vi "SWT_CarT_0722.vi"() -> ()   [LabVIEW 2013]
uses:
  <vilib>/Utility/error.llb/DialogType.ctl
  <vilib>/DAQmx/write.llb/DAQmx Write (Analog DBL 1Chan 1Samp).vi
  <vilib>/DAQmx/create/channels.llb/DAQmx Create Channel (AO-Voltage-Basic).vi
  <vilib>/DAQmx/miscellaneous.llb/DAQmx Fill In Error Info.vi
panel:
  in  "RFP exp":dbl=1.35
  in  "GFP exp":dbl=1.35
  in  "BF exp":dbl=1.35
  in  "WF aquare":bool
  out "in TBD":bool
  in  "TBD":bool
  in  "Next":bool=TRUE
  in  "Delete":bool
  in  "index(1~n)":i32=17 min=-1 max=43 step=1
  out "yn":i32=32
  out "y pose":dbl=-0.987708848659002 format="%.4g"
  out "xn":i32=44
  out "x pose":dbl=1.0289425462047794 format="%.4g"
  out "TBD num":dbl=12.0
  out "Cell num":i32=60
  out "Total num":i32=2025
  in  "Coordinate Path":path=path "D:/20230823/WF/result.xlsx"
  in  "d WF":dbl=1.35
  in  "y WF":dbl=-1.3212
  in  "x WF":dbl=-2.141
  in  "Init":bool=TRUE
  in  "scan test":bool
  in  "Reset":bool
  out "备份细胞坐标数组(X,Y)":i32[][](array[numeric])=[[11, 43, 478, 478, 1], [4, 41, 428, 428, 1], [24, 45, 343, 343, 1], [27, 38, 342, 342, 1], [27, 19, 311, 311, 1], [36, 19, 306, 306, 1], [10, 42, 296, 329, 1], [23, 28, 291, 291, 1], [15, 22, 283, 283, 1], [9, 32, 261, 261, 1], [24, 23, 252, 280, 1], [37, 36, 251, 251, 1], [11, 38, 246, 246, 1], [27, 6, 245, 245, 1], [28, 42, 240, 240, 1], [40, 39, 240, 267, 1], [16, 23, 230, 230, 1], [15, 40, 228, 228, 1], [27, 34, 227, 227, 1], [27, 13, 225, 225, 1], [10, 32, 222, 222, 1], [11, 20, 208, 231, 1], [23, 19, 208, 208, 1], [21, 13, 204, 226, 1], [25, 21, 199, 199, 1], [21, 1, 199, 199, 1], [29, 2, 197, 197, 1], [23, 35, 193, 215, 1], [23, 43, 189, 189, 1], [8, 13, 188, 188, 1], [30, 42, 188, 188, 1], [16, 18, 183, 183, 1], [29, 22, 183, 183, 1], [14, 41, 181, 181, 1], [9, 19, 180, 180, 1], [37, 37, 179, 179, 1], [42, 13, 176, 176, 1], [16, 39, 171, 171, 1], [30, 12, 170, 189, 1], [17, 26, 168, 168, 1], [8, 28, 168, 187, 1], [40, 26, 167, 167, 1], [42, 29, 159, 159, 1], [15, 8, 159, 159, 1], [27, 28, 158, 176, 1], [17, 6, 154, 154, 1], [26, 26, 154, 154, 1], [18, 32, 150, 167, 1], [36, 33, 150, 150, 1], [9, 22, 147, 147, 1], [40, 36, 147, 147, 1], [35, 13, 146, 146, 1], [27, 11, 146, 146, 1], [24, 34, 145, 161, 1], [34, 26, 143, 159, 1], [28, 19, 143, 143, 1], [10, 16, 142, 142, 1], [24, 28, 139, 155, 1], [17, 23, 139, 154, 1], [19, 11, 136, 136, 1], [20, 23, 135, 135, 1], [44, 39, 133, 133, 1], [12, 16, 133, 148, 1], [38, 37, 133, 133, 1], [3, 26, 133, 133, 1], [32, 17, 133, 133, 1], [25, 20, 133, 133, 1], [24, 9, 131, 146, 1], [10, 22, 127, 127, 1], [43, 26, 127, 127, 1], [19, 36, 127, 127, 1], [14, 25, 125, 125, 1], [30, 34, 125, 139, 1], [10, 39, 124, 138, 1], [38, 36, 124, 124, 1], [5, 28, 123, 123, 1], [6, 32, 121, 121, 1], [28, 23, 120, 120, 1], [35, 26, 120, 120, 1], [28, 24, 119, 119, 1], [37, 35, 118, 118, 1], [11, 17, 117, 130, 1], [31, 21, 117, 117, 1], [29, 45, 117, 117, 1], [37, 29, 117, 117, 1], [41, 37, 116, 116, 1], [8, 26, 115, 128, 1], [15, 42, 115, 128, 1], [27, 27, 115, 115, 1], [14, 37, 115, 128, 1], [19, 10, 112, 112, 1], [35, 17, 110, 110, 1], [29, 38, 110, 110, 1], [37, 22, 110, 122, 1], [38, 7, 110, 110, 1], [28, 8, 109, 109, 1], [43, 25, 108, 108, 1], [26, 6, 107, 107, 1], [37, 15, 107, 107, 1], [10, 20, 106, 106, 1], [17, 44, 106, 106, 1], [44, 1, 106, 106, 1], [31, 41, 106, 106, 1], [20, 33, 106, 117, 1], [38, 20, 105, 105, 1], [40, 28, 105, 105, 1], [16, 34, 105, 105, 1], [33, 35, 105, 105, 1], [19, 26, 105, 105, 1], [11, 31, 105, 105, 1], [42, 19, 105, 105, 1], [24, 22, 105, 105, 1], [38, 28, 104, 104, 1], [42, 44, 104, 104, 1], [29, 19, 104, 104, 1], [30, 36, 104, 115, 1], [27, 12, 104, 104, 1], [27, 32, 103, 103, 1], [14, 34, 103, 103, 1], [27, 35, 102, 102, 1], [13, 20, 102, 113, 1], [39, 23, 101, 101, 1], [25, 26, 101, 101, 1], [19, 25, 101, 101, 1], [17, 31, 100, 100, 1], [24, 38, 100, 111, 1], [30, 23, 99, 110, 1], [11, 24, 99, 110, 1], [7, 39, 98, 109, 1], [10, 13, 98, 98, 1], [30, 26, 97, 97, 1], [32, 26, 97, 97, 1], [28, 21, 96, 107, 1], [40, 1, 96, 107, 1], [42, 25, 95, 95, 1], [4, 20, 95, 95, 1], [24, 27, 95, 95, 1], [43, 39, 94, 94, 1], [24, 40, 93, 104, 1], [6, 24, 92, 92, 1], [44, 35, 91, 101, 1], [4, 23, 91, 91, 1], [27, 18, 91, 101, 1], [26, 23, 91, 101, 1], [6, 26, 91, 91, 1], [27, 25, 90, 100, 1], [13, 31, 90, 90, 1], [1, 23, 90, 90, 1], [36, 9, 90, 90, 1], [15, 29, 89, 89, 1], [30, 31, 89, 89, 1], [25, 27, 89, 89, 1], [27, 31, 88, 88, 1], [15, 17, 88, 88, 1], [41, 10, 88, 88, 1], [11, 16, 87, 97, 1], [11, 40, 87, 87, 1], [43, 42, 87, 87, 1], [9, 34, 86, 86, 1], [35, 27, 86, 86, 1], [6, 34, 85, 85, 1], [24, 1, 84, 84, 1], [42, 36, 84, 84, 1], [23, 23, 84, 84, 1], [35, 22, 83, 83, 1], [30, 1, 83, 83, 1], [29, 4, 83, 83, 1], [3, 33, 83, 83, 1], [45, 6, 83, 83, 1], [20, 32, 82, 91, 1], [41, 17, 82, 91, 1], [39, 4, 82, 82, 1], [31, 36, 81, 81, 1], [45, 16, 81, 81, 1], [19, 17, 81, 89, 1], [24, 4, 80, 80, 1], [19, 33, 80, 80, 1], [21, 28, 80, 89, 1], [15, 9, 80, 80, 1], [4, 31, 80, 80, 1], [22, 7, 80, 80, 1], [41, 19, 79, 79, 1], [26, 24, 79, 79, 1], [18, 38, 79, 79, 1], [45, 11, 78, 78, 1], [19, 7, 78, 78, 1], [22, 16, 78, 78, 1], [31, 11, 78, 78, 1], [35, 10, 77, 77, 1], [28, 33, 77, 77, 1], [15, 35, 76, 85, 1], [28, 32, 76, 85, 1], [39, 26, 75, 75, 1], [26, 16, 75, 83, 1], [20, 1, 75, 83, 1], [6, 44, 75, 75, 1], [15, 21, 75, 75, 1], [28, 25, 75, 83, 1], [17, 5, 74, 74, 1], [41, 33, 74, 74, 1], [41, 21, 74, 74, 1], [25, 29, 74, 74, 1], [25, 2, 73, 73, 1], [6, 40, 73, 73, 1], [20, 26, 73, 81, 1], [45, 23, 73, 73, 1], [40, 37, 72, 80, 1], [30, 21, 72, 72, 1], [34, 34, 72, 80, 1], [9, 33, 72, 80, 1], [11, 4, 71, 71, 1], [16, 40, 71, 79, 1], [44, 32, 70, 70, 1], [20, 40, 70, 78, 1], [26, 20, 70, 78, 1], [41, 36, 70, 78, 1], [23, 12, 69, 69, 1], [22, 26, 69, 77, 1], [45, 21, 68, 68, 1], [25, 32, 68, 68, 1], [5, 29, 67, 67, 1], [23, 31, 67, 74, 1], [7, 41, 67, 74, 1], [27, 1, 67, 67, 1], [23, 32, 66, 74, 1], [35, 32, 66, 66, 1], [25, 16, 66, 73, 1], [18, 41, 66, 73, 1], [43, 5, 65, 65, 1], [14, 17, 65, 72, 1], [21, 43, 65, 65, 1], [28, 3, 65, 65, 1], [21, 7, 64, 64, 1], [14, 21, 63, 70, 1], [19, 23, 63, 70, 1], [24, 32, 62, 62, 1], [16, 20, 61, 61, 1], [5, 38, 60, 60, 1], [22, 32, 59, 66, 1], [15, 34, 59, 59, 1], [11, 32, 57, 63, 1], [8, 44, 56, 63, 1], [34, 21, 55, 61, 1], [29, 35, 52, 58, 1]]
  out "missing":i32[][](array[numeric])
  out "缺失坐标数":i32
  in  "Period 2/min":dbl
  in  "Repeat 2":dbl
  in  "Interval/ms":dbl=10.0
  in  "Offste/V":dbl=-1.0
  in  "Frame rate/Hz":dbl=50.0
  in  "Offset2/V":dbl=0.804
  in  "Volume num":dbl=360.0
  in  "slice par stack":dbl=120.0
  in  "step/um":dbl=0.6
  out "细胞坐标数组(X,Y)":i32[][](array[numeric])=[[27, 34, 227, 227, 1], [21, 13, 204, 226, 1], [29, 2, 197, 197, 1], [30, 42, 188, 188, 1], [9, 22, 147, 147, 1], [6, 32, 121, 121, 1], [28, 8, 109, 109, 1], [14, 34, 103, 103, 1], [27, 35, 102, 102, 1], [41, 19, 79, 79, 1], [39, 26, 75, 75, 1], [6, 44, 75, 75, 1], [41, 21, 74, 74, 1], [20, 26, 73, 81, 1], [34, 34, 72, 80, 1], [11, 4, 71, 71, 1], [44, 32, 70, 70, 1], [20, 40, 70, 78, 1], [26, 20, 70, 78, 1], [41, 36, 70, 78, 1], [23, 12, 69, 69, 1], [22, 26, 69, 77, 1], [45, 21, 68, 68, 1], [25, 32, 68, 68, 1], [5, 29, 67, 67, 1], [23, 31, 67, 74, 1], [7, 41, 67, 74, 1], [27, 1, 67, 67, 1], [23, 32, 66, 74, 1], [35, 32, 66, 66, 1], [25, 16, 66, 73, 1], [18, 41, 66, 73, 1], [43, 5, 65, 65, 1], [14, 17, 65, 72, 1], [21, 43, 65, 65, 1], [28, 3, 65, 65, 1], [21, 7, 64, 64, 1], [14, 21, 63, 70, 1], [19, 23, 63, 70, 1], [24, 32, 62, 62, 1], [16, 20, 61, 61, 1], [5, 38, 60, 60, 1], [22, 32, 59, 66, 1], [15, 34, 59, 59, 1], [11, 32, 57, 63, 1], [8, 44, 56, 63, 1], [34, 21, 55, 61, 1], [29, 35, 52, 58, 1], [15, 40, 228, 228, 1], [26, 26, 154, 154, 1], [20, 23, 135, 135, 1], [24, 38, 100, 111, 1], [4, 41, 428, 428, 1], [24, 45, 343, 343, 1], [23, 43, 189, 189, 1], [18, 32, 150, 167, 1], [29, 45, 117, 117, 1], [19, 26, 105, 105, 1], [30, 36, 104, 115, 1], [41, 17, 82, 91, 1]]
  in  "x2 index":i32=41 min=1 max=45 step=1
  in  "y2 index":i32=41 min=1 max=45 step=1
  in  "y1 index":i32=1 min=1 max=45 step=1
  in  "x1 index":i32=5 min=1 max=45 step=1
  in  "y2":dbl=-1.7723000000000002 format="%.4f"
  in  "x2":dbl=0.7769500000000003 format="%.4f"
  in  "y1":dbl=1.811900000000001 format="%.4f"
  in  "x1":dbl=-2.4755499999999997 format="%.4f"
  in  "y to end":bool=TRUE
  in  "y to start":bool
  in  "x to end":bool=TRUE
  in  "x step forward":bool
  in  "x to start":bool=TRUE
  in  "x step backward":bool
  in  "y step backward":bool=TRUE
  in  "y step forward":bool
  out "芯片角点坐标":T1={"x1"=-2.4755499999999997, "y1"=1.811900000000001, "x2"=0.7769500000000003, "y2"=-1.7723000000000002, "x1 index"=5, "y1 index"=1, "x2 index"=41, "y2 index"=41, array2025x7[14175 elements], "missing"=[]}
  out "模板孔坐标数组":dbl[][](array[numeric])
  in  "Scanner":dbl(slide)=45.99999999999999 min=-50.0 max=150.0 step=1.0 scale=0.0..100.0
  out "finish":bool
  out "running":bool
  in  "Chanber num":dbl=17.0
  out "photo number":dbl
  in  "Period/min":dbl
  in  "Repeat":dbl=1.0
  in  "finish":bool=TRUE
  # "HUST WZF\n2023.08.20"
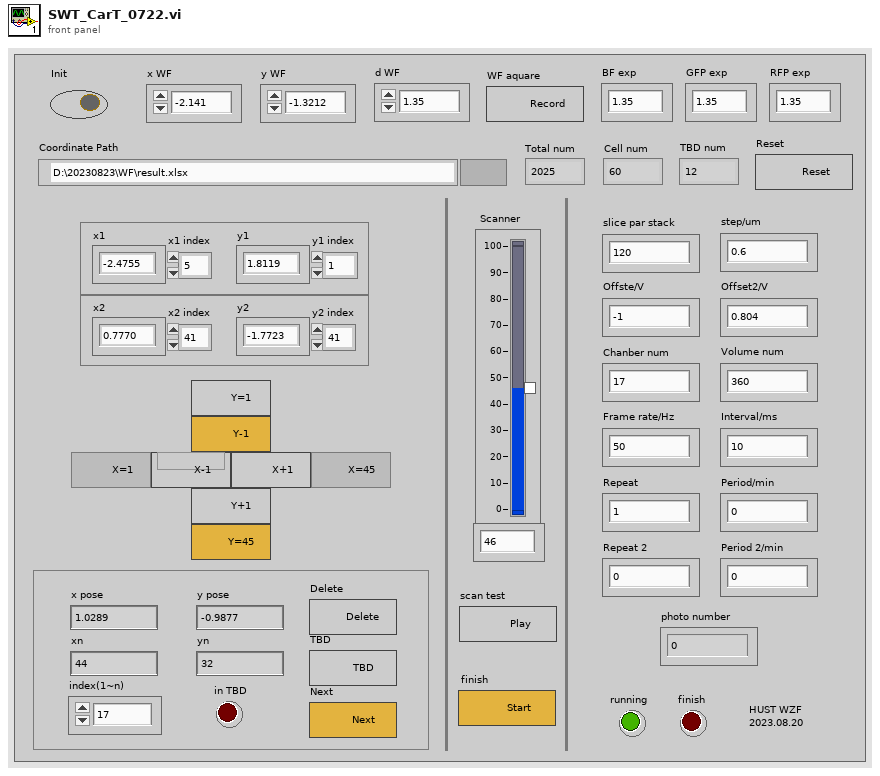
[diagram p1: front panel]
types:
  T1 = cluster{"x1":dbl, "y1":dbl, "x2":dbl, "y2":dbl, "x1 index":i32, "y1 index":i32, "x2 index":i32, "y2 index":i32, dbl[][], "missing":i32[][]}
  T2 = typedef "DialogType.ctl" = u16
  T3 = cluster{"x WF":dbl, "y WF":dbl, "d WF":dbl, "x1 index":i32, "y1 index":i32, "x2 index":i32, "y2 index":i32, dbl[][]}
  T4 = cluster{"y2":dbl, "y2":dbl, "y2":dbl, "y2":dbl, "x1 index":i32, "y1 index":i32, "x2 index":i32, "y2 index":i32, dbl[][], i32[][]}
  T5 = enum8{"Enabled", "Disabled", "Disabled and Grayed Out"}
  T6 = cluster{"x1":dbl, "y1":dbl, "x2":dbl, "y2":dbl, "x1 index":i32, "y1 index":i32, "x2 index":i32, "y2 index":i32, "模板孔坐标数组":dbl[][], "missing":i32[][]}
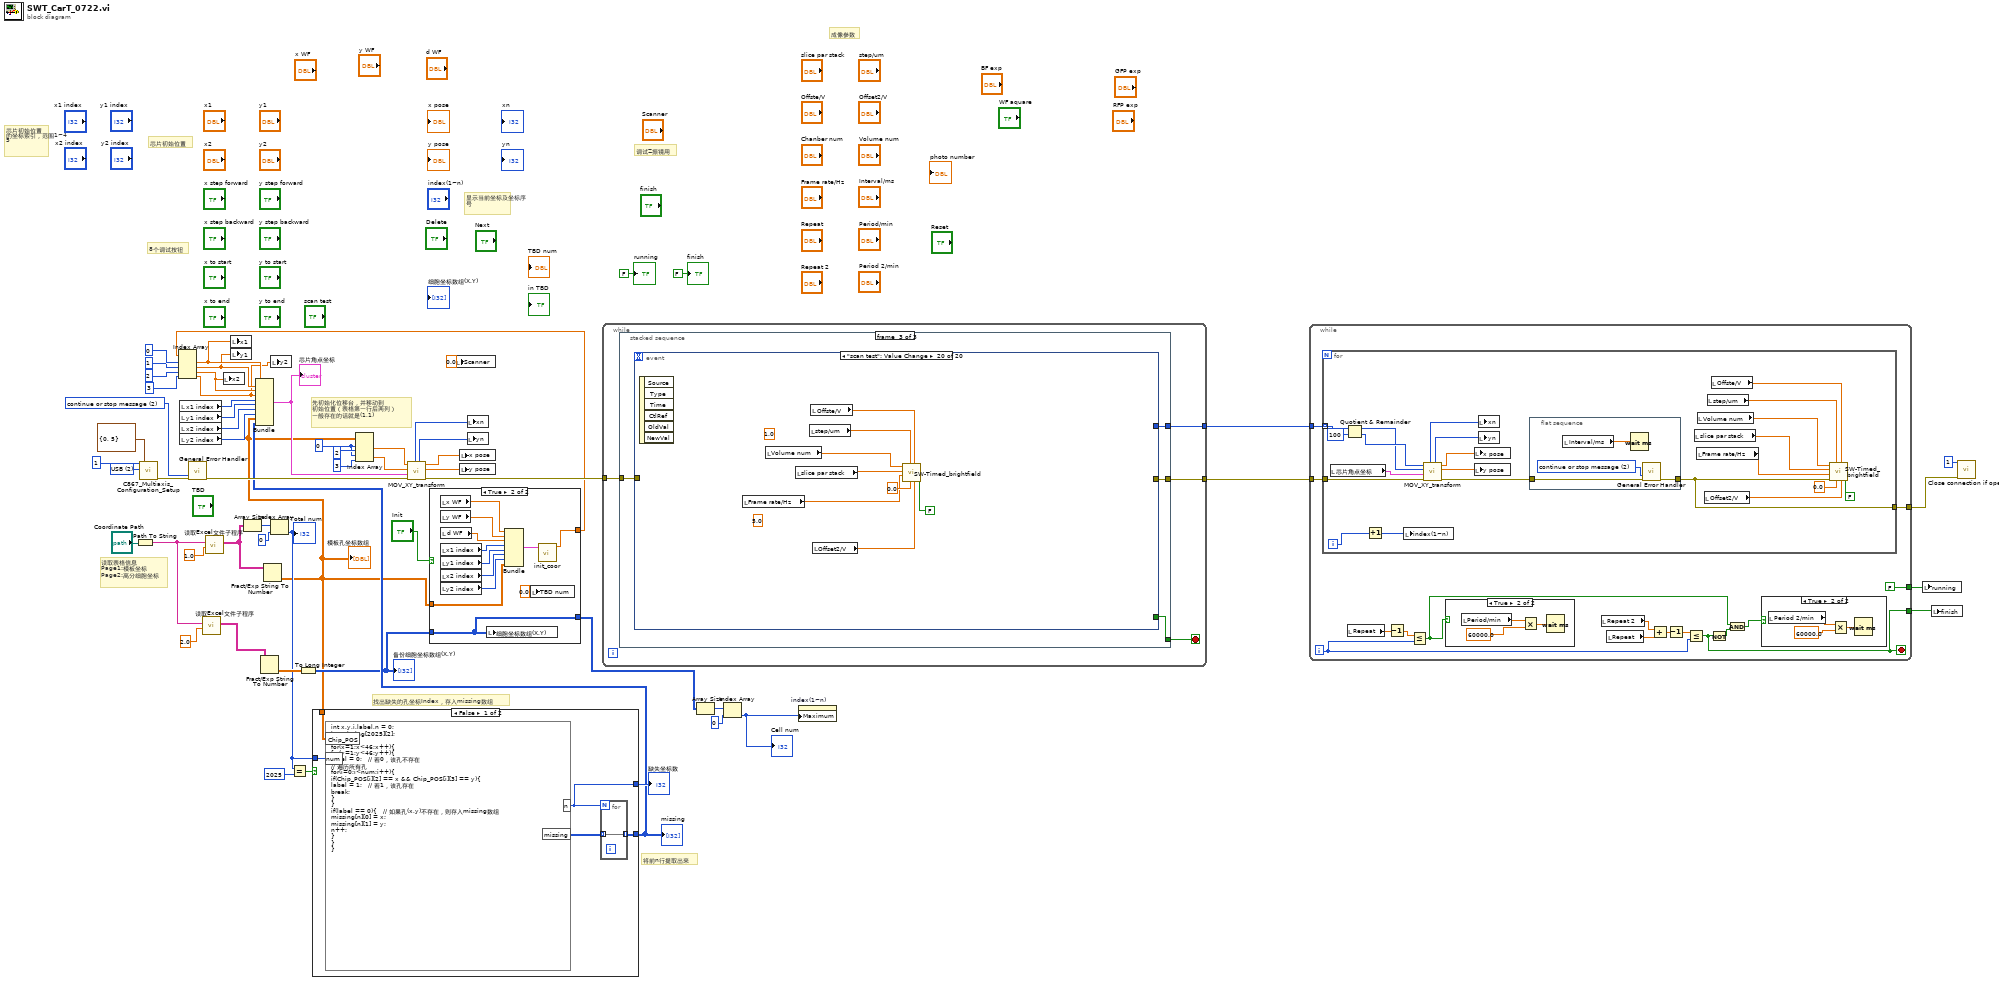
[diagram p0: block diagram]
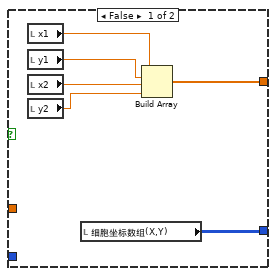
[diagram p2: hidden frame]
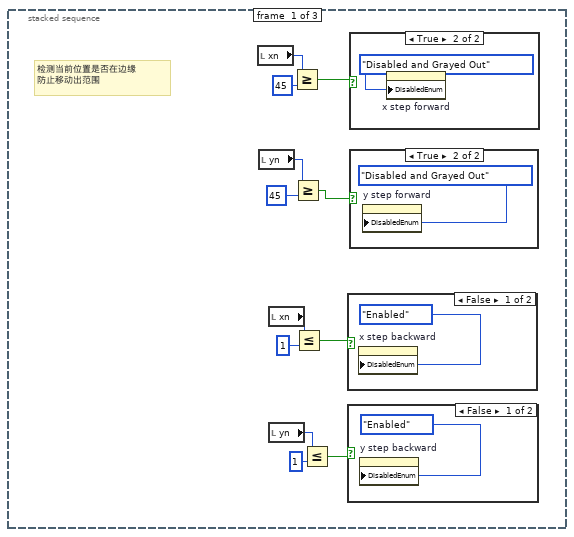
[diagram p5: hidden frame]
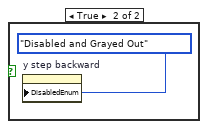
[diagram p6: hidden frame]
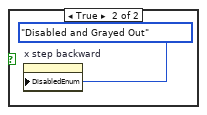
[diagram p7: hidden frame]
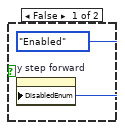
[diagram p8: hidden frame]
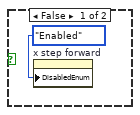
[diagram p9: hidden frame]
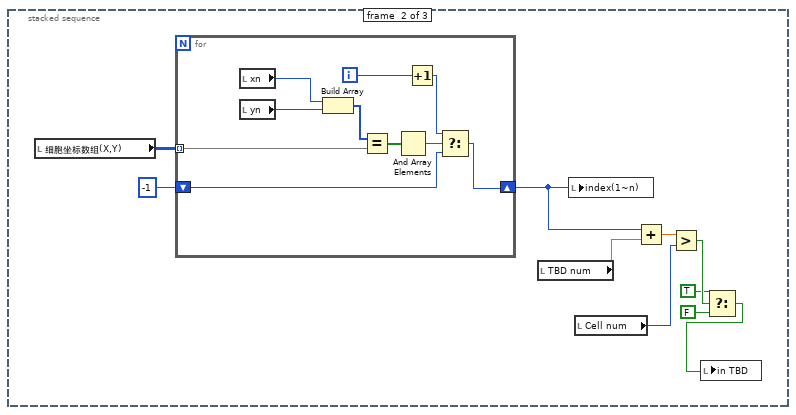
[diagram p10: hidden frame]
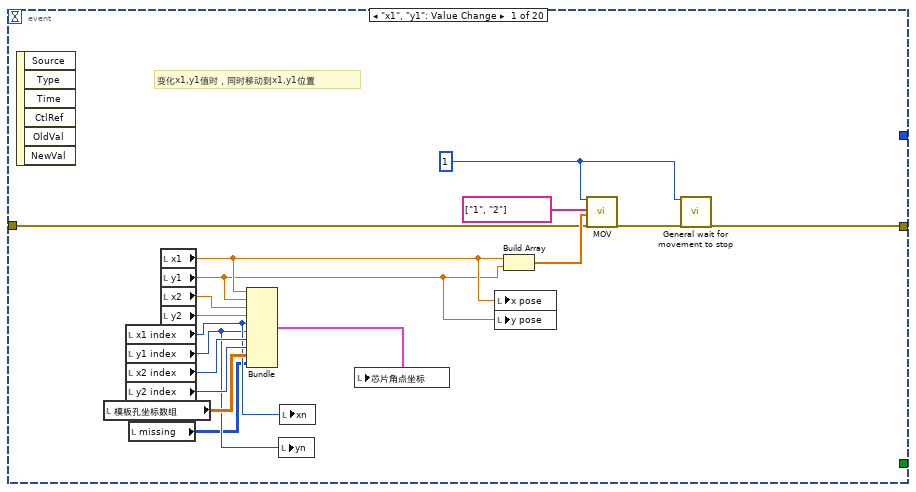
[diagram p11: hidden frame]
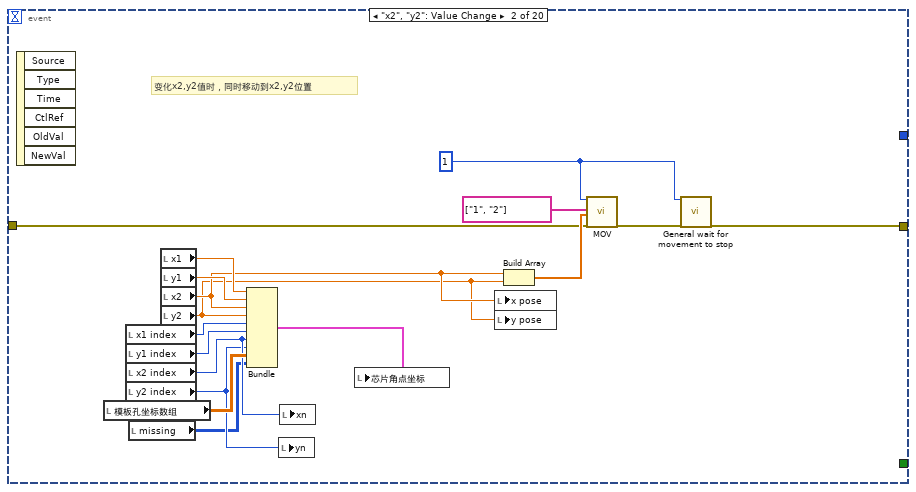
[diagram p12: hidden frame]
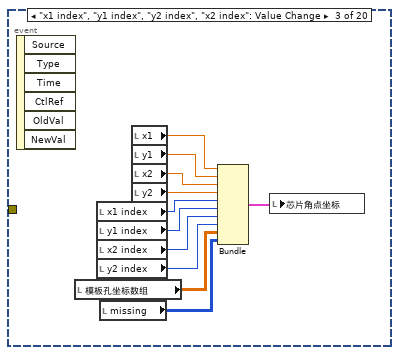
[diagram p13: hidden frame]
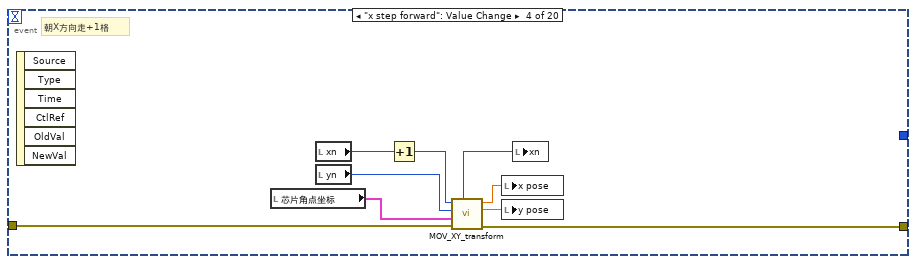
[diagram p14: hidden frame]
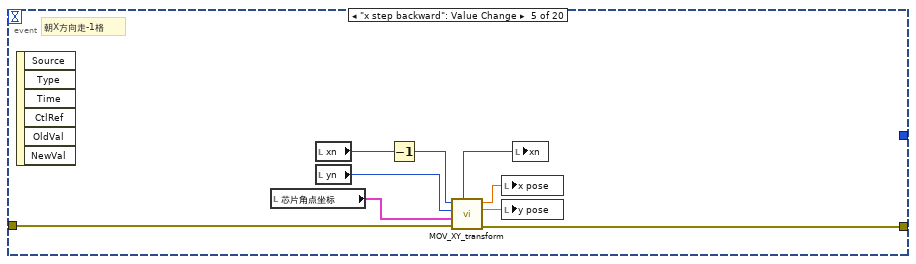
[diagram p15: hidden frame]
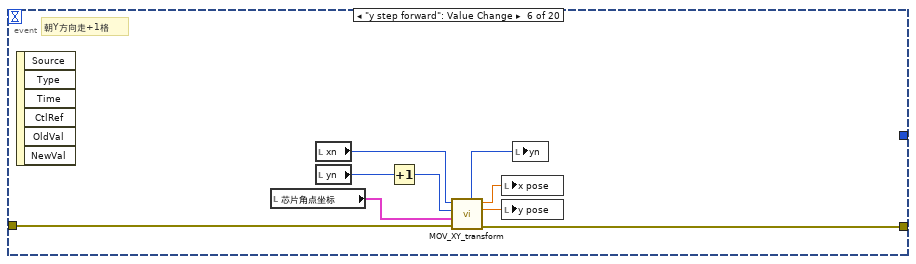
[diagram p16: hidden frame]
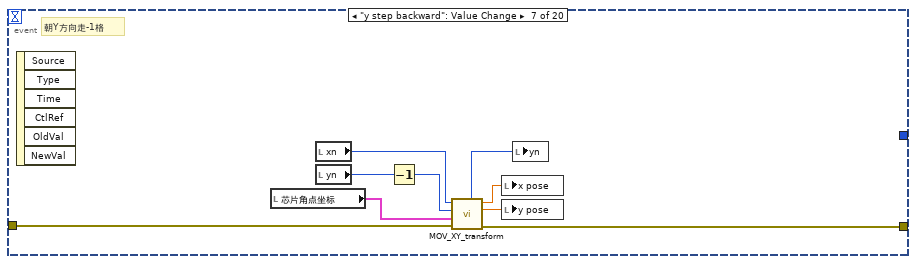
[diagram p17: hidden frame]
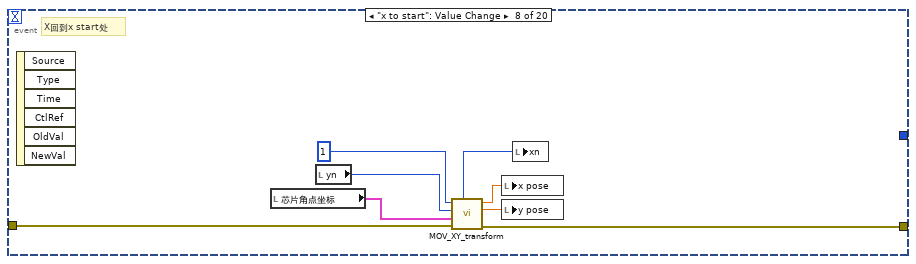
[diagram p18: hidden frame]
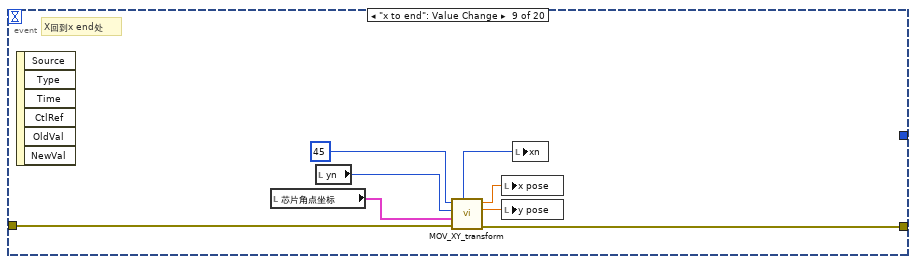
[diagram p19: hidden frame]
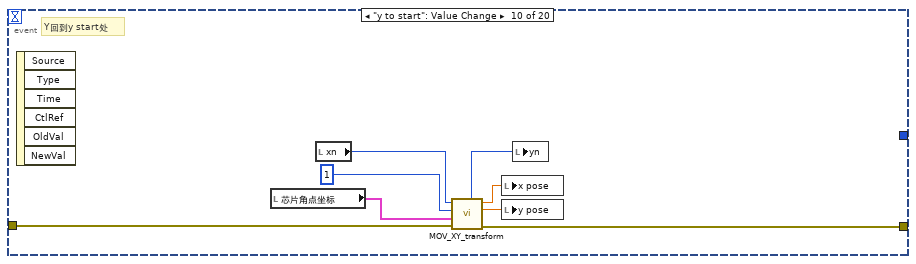
[diagram p20: hidden frame]
diagram:
  w18 = 0 ("索引 (行)")
  w53 = T2 2 items=["no dialog", "OK message", "continue or stop message", "OK message + warnings", "continue/stop + warnings"] ("type of dialog (OK msg:1)")
  w57 = u16 2 items=["RS232", "RS232 DaisyChain", "USB"] ("Interface")
  # "将前n行提取出来"
  # "找出缺失的孔坐标Index，存入missing数组"
  # "读取表格信息\nPage1:模板坐标\nPage2:高分细胞坐标"
  # "芯片初始位置\n的坐标索引，范围1~45"
  # "先初始化位移台，并移动到\n初始位置（表格第一行后两列）\n一般存在的话就是(1,1)"
  # "芯片初始位置"
  # "显示当前坐标及坐标序号"
  # "调试Z振镜用"
  # "8个调试按钮"
  # "成像参数"
  n1 = Path To String(path="Coordinate Path") -> (string=w39:string)
  n2 = call "C867_Multiaxis_Configuration_Setup.vi"("System no."=1, "Interface"=w57, "RS232 settings"=cluster{"Portnumber":i32, "Baudrate":u16} {"Portnumber"=0, "Baudrate"=5}) -> ("error out"=w54:errorcluster)  [unwired: 10 in, 6 out]
  n3 = local read "x1 index"() -> (w48:i32)
  n4 = local read "y1 index"() -> (w47:i32)
  n5 = local read "x2 index"() -> (w46:i32)
  n6 = local read "y2 index"() -> (w45:i32)
  n7 = call <vilib>:"General Error Handler.vi"("type of dialog (OK msg:1)"=w53, "error in (no error)"=w54) -> ("error out"=w52:errorcluster)  [unwired: 9 in, 4 out]
  n8 = call "读取Excel文件子程序.vi"("页"=2.0, "Filename"=w39) -> ("数据"=w42:string[][])  [unwired: 8 in, 1 out]
  n9 = call "读取Excel文件子程序.vi"("页"=1.0, "Filename"=w39) -> ("数据"=w43:string[][])  [unwired: 8 in, 1 out]
  n10 = Array Size(array=w43) -> (size(s)=w50:i32[])
  n11 = Fract/Exp String To Number(string=w42) -> (number=w37:dbl[][])  [unwired: 3 in, 1 out]
  n12 = Fract/Exp String To Number(string=w43) -> (number=w6:dbl[][])  [unwired: 3 in, 1 out]
  "模板孔坐标数组" <- w6
  n13 = Index Array(array=w50, index=0 ("索引")) -> (element=w34:i32)
  "Total num" <- w34
  n14 = Equal?(x=w34, y=2025) -> (x = y?=w36:bool)
  n15 = To Long Integer(number=w37) -> (32bit integer=w12:i32[][])
  "备份细胞坐标数组(X,Y)" <- w12
  n16 = case shown="False" w36 {
    tunnel: w6 -> [w65 _]
    tunnel: w34 -> [w64 _]
    tunnel: [w62 i32[][] []] -> w16
    tunnel: [w61 0] -> w23
    frame False {
      n17 = formula code="int x,y,i,label,n = 0;\nint missing[2025][2];\n\nfor(x=1;x<46;x++){\nfor(y=1;y<46;y++){\nlabel = 0;   // 若0，该孔不存在\n// 遍历所有孔\nfor(i=0;i<num;i++){\nif(Chip_POS[i][2] == x && Chip_POS[i][3] == y){\nlabel = 1;   // 若1，该孔存在\nbreak;\n}\n}\nif(label == 0){   // 如果孔(x,y)不存在，则存入missing数组\nmissing[n][0] = x;\nmissing[n][1] = y;\nn++;\n}\n}\n}"("Chip_POS"=w65, "num"=w64) -> ("missing"=w63:i32[][], "n"=w61:i32)
      n18 = for {
        N: w61 -> [_]
        tunnel: w63 -> [w66] mode=indexing
        tunnel: [w66] -> w62 mode=indexing
      }
    }
    frame True {
    }
  }
  "缺失坐标数" <- w23
  "missing" <- w16
  n19 = Index Array(array=w6, index (row) #1=w18, index (col) #1=2 ("禁用的索引 (列)"), index (row) #2=w18, index (col) #2=3 ("索引 (列)")) -> (element #1=w22:dbl, element #2=w19:dbl)
  n20 = case shown="True" "Init" {
    tunnel: w12 -> [_ w76]
    tunnel: [w70 w77] -> w11
    tunnel: w6 -> [_ w82]
    tunnel: [w69 w76] -> w1
    frame False {
      n21 = local read "x1"() -> (w74:dbl)
      n22 = local read "y1"() -> (w73:dbl)
      n23 = local read "x2"() -> (w72:dbl)
      n24 = local read "y2"() -> (w71:dbl)
      n25 = local read "细胞坐标数组(X,Y)"() -> (w69:i32[][])
      n26 = Build Array(w74, w73, w72, w71) -> (w70:dbl[])
    }
    frame True {
      n27 = local read "x WF"() -> (w81:dbl)
      n28 = local read "y WF"() -> (w80:dbl)
      n29 = local read "x1 index"() -> (w86:i32)
      n30 = local read "y1 index"() -> (w85:i32)
      n31 = local read "x2 index"() -> (w84:i32)
      n32 = local read "y2 index"() -> (w83:i32)
      n33 = local read "d WF"() -> (w79:dbl)
      n34 = local write "细胞坐标数组(X,Y)"(w76) -> ()
      n35 = Bundle("x WF"=w81, "y WF"=w80, "d WF"=w79, "x1 index"=w86, "y1 index"=w85, "x2 index"=w84, "y2 index"=w83, w82) -> (w78:T3)  [unwired: 1 in]
      n36 = local write "TBD num"(0.0 ("待定数")) -> ()
      n37 = call "init_coor.vi"("芯片角点坐标"=w78) -> ("x+y"=w77:dbl[])  [unwired: 10 in]
    }
  }
  n38 = Index Array(array=w11, index #1=0 ("index"), index #2=1 ("index"), index #3=2 ("index"), index #4=3 ("index")) -> (element #1=w5:dbl, element #2=w4:dbl, element #3=w3:dbl, element #4=w2:dbl)
  n39 = local write "x2"(w3) -> ()
  n40 = local write "x1"(w5) -> ()
  n41 = local write "y1"(w4) -> ()
  n42 = Bundle("y2"=w5, "y2"=w4, "y2"=w3, "y2"=w2, "x1 index"=w48, "y1 index"=w47, "x2 index"=w46, "y2 index"=w45, w6, w16) -> (w20:T4)  [unwired: 1 in]
  "芯片角点坐标" <- w20
  n43 = local write "y2"(w2) -> ()
  n44 = call "MOV_XY_transform.vi"("error in"=w52, "芯片角点坐标"=w20, "y index"=w19, "x index"=w22) -> ("error out"=w60:errorcluster, "Y当前位置(mm)"=w58:dbl, "X当前位置(mm)"=w59:dbl, "Y实际坐标数"=w14:i32, "X实际坐标数"=w15:i32)  [unwired: 1 in]
  n45 = local write "Scanner"(0.0 ("振镜")) -> ()
  n46 = local write "x pose"(w59) -> ()
  n47 = local write "y pose"(w58) -> ()
  n48 = local write "xn"(w15) -> ()
  n49 = local write "yn"(w14) -> ()
  n50 = while {
    tunnel: w60 -> [w87]
    tunnel: [w90] -> w30
    tunnel: [w88] -> w29
    stop <- w89 stop-if-true
    n51 = stacked-sequence {
      tunnel: [_ _ w134] -> w90
      tunnel: [_ _ w133] -> w89
      tunnel: [_ _ w132] -> w88
      tunnel: w87 -> [_ _ w131]
      frame #0 {
        # "检测当前位置是否在边缘\n防止移动出范围"
        n52 = local read "xn"() -> (w97:i32)
        n53 = local read "yn"() -> (w98:i32)
        n54 = local read "xn"() -> (w101:i32)
        n55 = local read "yn"() -> (w102:i32)
        n56 = Greater Or Equal?(x=w97, y=45) -> (x >= y?=w93:bool)
        n57 = Greater Or Equal?(x=w98, y=45) -> (x >= y?=w94:bool)
        n58 = Less Or Equal?(x=w101, y=1) -> (x <= y?=w92:bool)
        n59 = Less Or Equal?(x=w102, y=1) -> (x <= y?=w91:bool)
        n60 = case shown="False" w92 {
          frame False {
            n61 = property on="x step backward" class="Bool"("DisabledEnum"=T5."Enabled" ("禁用")) -> ()  [unwired: 2 in, 2 out]
          }
          frame True {
            n62 = property on="x step backward" class="Bool"("DisabledEnum"=T5."Disabled and Grayed Out" ("禁用")) -> ()  [unwired: 2 in, 2 out]
          }
        }
        n63 = case shown="False" w91 {
          frame False {
            n64 = property on="y step backward" class="Bool"("DisabledEnum"=T5."Enabled" ("禁用")) -> ()  [unwired: 2 in, 2 out]
          }
          frame True {
            n65 = property on="y step backward" class="Bool"("DisabledEnum"=T5."Disabled and Grayed Out" ("禁用")) -> ()  [unwired: 2 in, 2 out]
          }
        }
        n66 = case shown="True" w93 {
          frame False {
            n67 = property on="x step forward" class="Bool"("DisabledEnum"=T5."Enabled" ("禁用")) -> ()  [unwired: 2 in, 2 out]
          }
          frame True {
            n68 = property on="x step forward" class="Bool"("DisabledEnum"=T5."Disabled and Grayed Out" ("禁用")) -> ()  [unwired: 2 in, 2 out]
          }
        }
        n69 = case shown="True" w94 {
          frame False {
            n70 = property on="y step forward" class="Bool"("DisabledEnum"=T5."Enabled" ("禁用")) -> ()  [unwired: 2 in, 2 out]
          }
          frame True {
            n71 = property on="y step forward" class="Bool"("DisabledEnum"=T5."Disabled and Grayed Out" ("禁用")) -> ()  [unwired: 2 in, 2 out]
          }
        }
      }
      frame #1 {
        n72 = local read "细胞坐标数组(X,Y)"() -> (w120:i32[][])
        n73 = for {
          tunnel: w120 -> [w130] mode=indexing
          shift-right: [w121] -> w118
          shift-left: -1 ("当前细胞(1~n)") -> [w122]
          i -> [w124]
          n74 = local read "xn"() -> (w129:i32)
          n75 = local read "yn"() -> (w128:i32)
          n76 = Build Array(w129, w128) -> (w127:i32[])
          n77 = Equal?(x=w127, y=w130) -> (x = y?=w126:bool[])
          n78 = And Array Elements(Boolean array=w126) -> (logical AND=w125:bool)
          n79 = Increment(x=w124) -> (x+1=w123:i32)
          n80 = Select(t=w123, s=w125, f=w122) -> (s? t:f=w121:i32)
        }
        n81 = local read "TBD num"() -> (w117:dbl)
        n82 = local write "index(1~n)"(w118) -> ()
        n83 = local read "Cell num"() -> (w115:i32)
        n84 = Add(x=w118, y=w117) -> (x+y=w116:dbl)
        n85 = Greater?(x=w116, y=w115) -> (0:w114:bool)
        n86 = Select(t=TRUE, s=w114, f=FALSE) -> (s? t:f=w113:bool)
        n87 = local write "in TBD"(w113) -> ()
      }
      frame #2 {
        n88 = event shown="[19] \"scan test\": Value Change" {
          selector: _ -> [_ _ _ _ _ _ _ _ _ _ _ _ _ _ _ _ _ _ _ _]
          dyn-events: _ -> [_ _ _ _ _ _ _ _ _ _ _ _ _ _ _ _ _ _ _ _]
          timeout: _ -> [_ _ _ _ _ _ _ _ _ _ _ _ _ _ _ _ _ _ _ _]
          tunnel: w131 -> [w138 w159 _ w188 w197 w206 w215 w223 w231 w239 w247 w254 w277 w297 w331 _ _ _ w398 _]
          tunnel: [w139 w160 _ w187 w196 w205 w214 w222 w230 w238 w246 w253 w276 w296 w330 _ _ _ w398 _] -> w134
          tunnel: [_ _ _ _ _ _ _ _ _ _ _ _ _ _ _ _ _ _ TRUE ("finish compensation") _] -> w133
          tunnel: [_ _ _ _ _ _ _ _ _ _ _ _ _ _ _ _ _ _ w395 _] -> w132
          event "x1", "y1": Value Change {
            w145 = 1 ("System no.")
            # "变化x1,y1值时，同时移动到x1,y1位置"
            n89 = event-data() -> ()  [unwired: 1 in, 6 out]
            n90 = local read "模板孔坐标数组"() -> (w146:dbl[][])
            n91 = local read "x1 index"() -> (w141:i32)
            n92 = local read "y1 index"() -> (w140:i32)
            n93 = local read "x2 index"() -> (w150:i32)
            n94 = local read "y2 index"() -> (w151:i32)
            n95 = local read "missing"() -> (w135:i32[][])
            n96 = local read "x1"() -> (w137:dbl)
            n97 = local read "y1"() -> (w136:dbl)
            n98 = local read "x2"() -> (w148:dbl)
            n99 = local read "y2"() -> (w149:dbl)
            n100 = Bundle("x1"=w137, "y1"=w136, "x2"=w148, "y2"=w149, "x1 index"=w141, "y1 index"=w140, "x2 index"=w150, "y2 index"=w151, "模板孔坐标数组"=w146, "missing"=w135) -> (w147:T6)  [unwired: 1 in]
            n101 = local write "yn"(w140) -> ()
            n102 = local write "xn"(w141) -> ()
            n103 = local write "芯片角点坐标"(w147) -> ()
            n104 = local write "x pose"(w137) -> ()
            n105 = local write "y pose"(w136) -> ()
            n106 = Build Array(w137, w136) -> (w143:dbl[])
            n107 = call "MOV.vi"("System no."=w145, "Axes to move"=string[] ["1", "2"], "Position values"=w143, "error in"=w138) -> ("error out"=w142:errorcluster)  [unwired: 15 in]
            n108 = call "General wait for movement to stop.vi"("System no."=w145, "error in"=w142) -> ("error out"=w139:errorcluster)  [unwired: 16 in, 1 out]
          }
          event "x2", "y2": Value Change {
            w166 = 1 ("System no.")
            # "变化x2,y2值时，同时移动到x2,y2位置"
            n109 = event-data() -> ()  [unwired: 1 in, 6 out]
            n110 = local read "模板孔坐标数组"() -> (w167:dbl[][])
            n111 = local read "x1 index"() -> (w162:i32)
            n112 = local read "y1 index"() -> (w161:i32)
            n113 = local read "x2 index"() -> (w156:i32)
            n114 = local read "y2 index"() -> (w155:i32)
            n115 = local read "missing"() -> (w152:i32[][])
            n116 = local read "x1"() -> (w158:dbl)
            n117 = local read "y1"() -> (w157:dbl)
            n118 = local read "x2"() -> (w154:dbl)
            n119 = local read "y2"() -> (w153:dbl)
            n120 = Bundle("x1"=w158, "y1"=w157, "x2"=w154, "y2"=w153, "x1 index"=w162, "y1 index"=w161, "x2 index"=w156, "y2 index"=w155, "模板孔坐标数组"=w167, "missing"=w152) -> (w168:T6)  [unwired: 1 in]
            n121 = local write "yn"(w155) -> ()
            n122 = local write "xn"(w156) -> ()
            n123 = local write "芯片角点坐标"(w168) -> ()
            n124 = local write "x pose"(w154) -> ()
            n125 = local write "y pose"(w153) -> ()
            n126 = Build Array(w154, w153) -> (w164:dbl[])
            n127 = call "MOV.vi"("System no."=w166, "Axes to move"=string[] ["1", "2"], "Position values"=w164, "error in"=w159) -> ("error out"=w163:errorcluster)  [unwired: 15 in]
            n128 = call "General wait for movement to stop.vi"("System no."=w166, "error in"=w163) -> ("error out"=w160:errorcluster)  [unwired: 16 in, 1 out]
          }
          event "x1 index", "y1 index", "y2 index", "x2 index": Value Change {
            n129 = event-data() -> ()  [unwired: 1 in, 6 out]
            n130 = local read "模板孔坐标数组"() -> (w170:dbl[][])
            n131 = local read "x1 index"() -> (w176:i32)
            n132 = local read "y1 index"() -> (w177:i32)
            n133 = local read "x2 index"() -> (w178:i32)
            n134 = local read "y2 index"() -> (w179:i32)
            n135 = local read "missing"() -> (w169:i32[][])
            n136 = local read "x1"() -> (w172:dbl)
            n137 = local read "y1"() -> (w173:dbl)
            n138 = local read "x2"() -> (w174:dbl)
            n139 = local read "y2"() -> (w175:dbl)
            n140 = Bundle("x1"=w172, "y1"=w173, "x2"=w174, "y2"=w175, "x1 index"=w176, "y1 index"=w177, "x2 index"=w178, "y2 index"=w179, "模板孔坐标数组"=w170, "missing"=w169) -> (w171:T6)  [unwired: 1 in]
            n141 = local write "芯片角点坐标"(w171) -> ()
          }
          event "x step forward": Value Change {
            # "朝X方向走+1格"
            n142 = event-data() -> ()  [unwired: 1 in, 6 out]
            n143 = local read "芯片角点坐标"() -> (w184:T1)
            n144 = local read "xn"() -> (w186:i32)
            n145 = local read "yn"() -> (w185:i32)
            n146 = Increment(x=w186) -> (x+1=w183:i32)
            n147 = call "MOV_XY_transform.vi"("error in"=w188, "芯片角点坐标"=w184, "y index"=w185, "x index"=w183) -> ("error out"=w187:errorcluster, "Y当前位置(mm)"=w182:dbl, "X当前位置(mm)"=w181:dbl, "X实际坐标数"=w180:i32)  [unwired: 1 in, 1 out]
            n148 = local write "x pose"(w181) -> ()
            n149 = local write "y pose"(w182) -> ()
            n150 = local write "xn"(w180) -> ()
          }
          event "x step backward": Value Change {
            # "朝X方向走-1格"
            n151 = event-data() -> ()  [unwired: 1 in, 6 out]
            n152 = local read "芯片角点坐标"() -> (w193:T1)
            n153 = local read "xn"() -> (w195:i32)
            n154 = local read "yn"() -> (w194:i32)
            n155 = Decrement(x=w195) -> (x-1=w192:i32)
            n156 = call "MOV_XY_transform.vi"("error in"=w197, "芯片角点坐标"=w193, "y index"=w194, "x index"=w192) -> ("error out"=w196:errorcluster, "Y当前位置(mm)"=w191:dbl, "X当前位置(mm)"=w190:dbl, "X实际坐标数"=w189:i32)  [unwired: 1 in, 1 out]
            n157 = local write "x pose"(w190) -> ()
            n158 = local write "y pose"(w191) -> ()
            n159 = local write "xn"(w189) -> ()
          }
          event "y step forward": Value Change {
            # "朝Y方向走+1格"
            n160 = event-data() -> ()  [unwired: 1 in, 6 out]
            n161 = local read "芯片角点坐标"() -> (w204:T1)
            n162 = local read "xn"() -> (w201:i32)
            n163 = local read "yn"() -> (w200:i32)
            n164 = Increment(x=w200) -> (x+1=w199:i32)
            n165 = call "MOV_XY_transform.vi"("error in"=w206, "芯片角点坐标"=w204, "y index"=w199, "x index"=w201) -> ("error out"=w205:errorcluster, "Y当前位置(mm)"=w203:dbl, "X当前位置(mm)"=w202:dbl, "Y实际坐标数"=w198:i32)  [unwired: 1 in, 1 out]
            n166 = local write "x pose"(w202) -> ()
            n167 = local write "y pose"(w203) -> ()
            n168 = local write "yn"(w198) -> ()
          }
          event "y step backward": Value Change {
            # "朝Y方向走-1格"
            n169 = event-data() -> ()  [unwired: 1 in, 6 out]
            n170 = local read "芯片角点坐标"() -> (w213:T1)
            n171 = local read "xn"() -> (w210:i32)
            n172 = local read "yn"() -> (w209:i32)
            n173 = Decrement(x=w209) -> (x-1=w208:i32)
            n174 = call "MOV_XY_transform.vi"("error in"=w215, "芯片角点坐标"=w213, "y index"=w208, "x index"=w210) -> ("error out"=w214:errorcluster, "Y当前位置(mm)"=w212:dbl, "X当前位置(mm)"=w211:dbl, "Y实际坐标数"=w207:i32)  [unwired: 1 in, 1 out]
            n175 = local write "x pose"(w211) -> ()
            n176 = local write "y pose"(w212) -> ()
            n177 = local write "yn"(w207) -> ()
          }
          event "x to start": Value Change {
            # "X回到x start处"
            n178 = event-data() -> ()  [unwired: 1 in, 6 out]
            n179 = local read "芯片角点坐标"() -> (w221:T1)
            n180 = local read "yn"() -> (w218:i32)
            n181 = call "MOV_XY_transform.vi"("error in"=w223, "芯片角点坐标"=w221, "y index"=w218, "x index"=1) -> ("error out"=w222:errorcluster, "Y当前位置(mm)"=w220:dbl, "X当前位置(mm)"=w219:dbl, "X实际坐标数"=w216:i32)  [unwired: 1 in, 1 out]
            n182 = local write "x pose"(w219) -> ()
            n183 = local write "y pose"(w220) -> ()
            n184 = local write "xn"(w216) -> ()
          }
          event "x to end": Value Change {
            # "X回到x end处"
            n185 = event-data() -> ()  [unwired: 1 in, 6 out]
            n186 = local read "芯片角点坐标"() -> (w229:T1)
            n187 = local read "yn"() -> (w226:i32)
            n188 = call "MOV_XY_transform.vi"("error in"=w231, "芯片角点坐标"=w229, "y index"=w226, "x index"=45) -> ("error out"=w230:errorcluster, "Y当前位置(mm)"=w228:dbl, "X当前位置(mm)"=w227:dbl, "X实际坐标数"=w224:i32)  [unwired: 1 in, 1 out]
            n189 = local write "x pose"(w227) -> ()
            n190 = local write "y pose"(w228) -> ()
            n191 = local write "xn"(w224) -> ()
          }
          event "y to start": Value Change {
            # "Y回到y start处"
            n192 = event-data() -> ()  [unwired: 1 in, 6 out]
            n193 = local read "芯片角点坐标"() -> (w237:T1)
            n194 = local read "xn"() -> (w234:i32)
            n195 = call "MOV_XY_transform.vi"("error in"=w239, "芯片角点坐标"=w237, "y index"=1, "x index"=w234) -> ("error out"=w238:errorcluster, "Y当前位置(mm)"=w236:dbl, "X当前位置(mm)"=w235:dbl, "Y实际坐标数"=w232:i32)  [unwired: 1 in, 1 out]
            n196 = local write "x pose"(w235) -> ()
            n197 = local write "y pose"(w236) -> ()
            n198 = local write "yn"(w232) -> ()
          }
          event "y to end": Value Change {
            # "Y回到y end处"
            n199 = event-data() -> ()  [unwired: 1 in, 6 out]
            n200 = local read "芯片角点坐标"() -> (w245:T1)
            n201 = local read "xn"() -> (w242:i32)
            n202 = call "MOV_XY_transform.vi"("error in"=w247, "芯片角点坐标"=w245, "y index"=45, "x index"=w242) -> ("error out"=w246:errorcluster, "Y当前位置(mm)"=w244:dbl, "X当前位置(mm)"=w243:dbl, "Y实际坐标数"=w240:i32)  [unwired: 1 in, 1 out]
            n203 = local write "x pose"(w243) -> ()
            n204 = local write "y pose"(w244) -> ()
            n205 = local write "yn"(w240) -> ()
          }
          event "index(1~n)": Value Change {
            n206 = event-data() -> ()  [unwired: 1 in, 6 out]
            n207 = local read "Cell num"() -> (w252:i32)
            n208 = local read "index(1~n)"() -> (w251:i32)
            n209 = Less Or Equal?(x=w251, y=w252) -> (x <= y?=w248:bool)
            n210 = Greater Than 0?(x=w251) -> (x > 0?=w249:bool)
            n211 = And(x=w249, y=w248) -> (x .and. y?=w250:bool)
            n212 = case shown="True" w250 {
              tunnel: w254 -> [w255 w266]
              tunnel: [w255 w265] -> w253
              tunnel: w251 -> [_ w259]
              frame False {
              }
              frame True {
                # "0列：X\n1列：Y"
                n213 = local read "细胞坐标数组(X,Y)"() -> (w269:i32[][])
                n214 = Decrement(x=w259) -> (x-1=w258:i32)
                n215 = local read "芯片角点坐标"() -> (w264:T1)
                n216 = Index Array(array=w269, index (row) #1=w258, index (col) #1=0 ("禁用的索引 (列)"), index (row) #2=w258, index (col) #2=1 ("禁用的索引 (列)")) -> (element #1=w260:i32, element #2=w261:i32)
                n217 = call "MOV_XY_transform.vi"("error in"=w266, "芯片角点坐标"=w264, "y index"=w261, "x index"=w260) -> ("error out"=w265:errorcluster, "Y当前位置(mm)"=w262:dbl, "X当前位置(mm)"=w263:dbl, "Y实际坐标数"=w256:i32, "X实际坐标数"=w257:i32)  [unwired: 1 in]
                n218 = local write "xn"(w257) -> ()
                n219 = local write "yn"(w256) -> ()
                n220 = local write "x pose"(w263) -> ()
                n221 = local write "y pose"(w262) -> ()
              }
            }
          }
          event "Next": Value Change {
            n222 = event-data() -> ()  [unwired: 1 in, 1 out]
            n223 = local read "index(1~n)"() -> (w271:i32)
            n224 = local read "Cell num"() -> (w275:i32)
            n225 = Increment(x=w271) -> (x+1=w270:i32)
            n226 = local write "index(1~n)"(w270) -> ()
            n227 = Less Or Equal?(x=w270, y=w275) -> (x <= y?=w272:bool)
            n228 = Greater Than 0?(x=w270) -> (x > 0?=w273:bool)
            n229 = And(x=w273, y=w272) -> (x .and. y?=w274:bool)
            n230 = case shown="True" w274 {
              tunnel: w277 -> [w278 w289]
              tunnel: [w278 w288] -> w276
              tunnel: w270 -> [_ w282]
              frame False {
              }
              frame True {
                # "0列：X\n1列：Y"
                n231 = local read "细胞坐标数组(X,Y)"() -> (w292:i32[][])
                n232 = Decrement(x=w282) -> (x-1=w281:i32)
                n233 = local read "芯片角点坐标"() -> (w287:T1)
                n234 = Index Array(array=w292, index (row) #1=w281, index (col) #1=0 ("禁用的索引 (列)"), index (row) #2=w281, index (col) #2=1 ("禁用的索引 (列)")) -> (element #1=w283:i32, element #2=w284:i32)
                n235 = call "MOV_XY_transform.vi"("error in"=w289, "芯片角点坐标"=w287, "y index"=w284, "x index"=w283) -> ("error out"=w288:errorcluster, "Y当前位置(mm)"=w285:dbl, "X当前位置(mm)"=w286:dbl, "Y实际坐标数"=w279:i32, "X实际坐标数"=w280:i32)  [unwired: 1 in]
                n236 = local write "xn"(w280) -> ()
                n237 = local write "yn"(w279) -> ()
                n238 = local write "x pose"(w286) -> ()
                n239 = local write "y pose"(w285) -> ()
              }
            }
          }
          event "Delete": Value Change {
            n240 = event-data() -> ()  [unwired: 1 in, 6 out]
            n241 = local read "Cell num"() -> (w295:i32)
            n242 = local read "index(1~n)"() -> (w294:i32)
            n243 = Equal?(x=w294, y=w295) -> (x = y?=w293:bool)
            n244 = Greater Than 0?(x=w294) -> (x > 0?=w298:bool)
            n245 = case shown="True" w298 {
              tunnel: w294 -> [_ w320]
              tunnel: w297 -> [w299 w314]
              tunnel: [w299 w313] -> w296
              tunnel: w293 -> [_ w307]
              frame False {
              }
              frame True {
                n246 = local read "细胞坐标数组(X,Y)"() -> (w322:i32[][])
                n247 = Decrement(x=w320) -> (x-1=w304:i32)
                n248 = local read "芯片角点坐标"() -> (w312:T1)
                n249 = Decrement(x=w304) -> (x-1=w305:i32)
                n250 = Select(t=w305, s=w307, f=w304) -> (s? t:f=w306:i32)
                n251 = Delete From Array(array=w322, index (row)=w304) -> (array with subset deleted=w315:i32[][])  [unwired: 2 in, 1 out]
                n252 = Array Size(array=w315) -> (size(s)=w324:i32[])
                n253 = local write "细胞坐标数组(X,Y)"(w315) -> ()
                n254 = Index Array(array=w315, index (row) #1=w306, index (col) #1=0 ("禁用的索引 (列)"), index (row) #2=w306, index (col) #2=1 ("禁用的索引 (列)")) -> (element #1=w316:i32, element #2=w317:i32)
                n255 = Index Array(array=w324, index=0 ("索引")) -> (element=w321:i32)
                n256 = property on="index(1~n)" class="DigNum (strict)"("Maximum"=w321) -> ()  [unwired: 2 in, 2 out]
                n257 = local write "Cell num"(w321) -> ()
                n258 = call "MOV_XY_transform.vi"("error in"=w314, "芯片角点坐标"=w312, "y index"=w317, "x index"=w316) -> ("error out"=w313:errorcluster, "Y当前位置(mm)"=w308:dbl, "X当前位置(mm)"=w309:dbl, "Y实际坐标数"=w310:i32, "X实际坐标数"=w311:i32)  [unwired: 1 in]
                n259 = local read "TBD num"() -> (w300:dbl)
                n260 = local write "x pose"(w309) -> ()
                n261 = local write "y pose"(w308) -> ()
                n262 = local read "in TBD"() -> (w303:bool)
                n263 = local write "xn"(w311) -> ()
                n264 = local write "yn"(w310) -> ()
                n265 = Decrement(x=w300) -> (x-1=w301:dbl)
                n266 = Select(t=w301, s=w303, f=w300) -> (s? t:f=w302:dbl)
                n267 = local write "TBD num"(w302) -> ()
              }
            }
          }
          event "TBD": Value Change {
            n268 = event-data() -> ()  [unwired: 1 in, 6 out]
            n269 = local read "Cell num"() -> (w329:i32)
            n270 = local read "index(1~n)"() -> (w328:i32)
            n271 = Less?(x=w328, y=w329) -> (x < y?=w326:bool)
            n272 = Greater Than 0?(x=w328) -> (x > 0?=w327:bool)
            n273 = And(x=w327, y=w326) -> (x .and. y?=w325:bool)
            n274 = case shown="True" w325 {
              tunnel: w328 -> [_ w354]
              tunnel: w331 -> [w332 w349]
              tunnel: [w332 w348] -> w330
              frame False {
              }
              frame True {
                n275 = local read "细胞坐标数组(X,Y)"() -> (w342:i32[][])
                n276 = Decrement(x=w354) -> (x-1=w341:i32)
                n277 = local read "芯片角点坐标"() -> (w347:T1)
                n278 = Array Subset(array=w342, index (row)=w341, length (row)=1 ("length")) -> (w338:i32[][])  [unwired: 2 in]
                n279 = Delete From Array(array=w342, index (row)=w341) -> (array with subset deleted=w339:i32[][])  [unwired: 2 in, 1 out]
                n280 = Insert Into Array(array=w339, new element=w338) -> (w337:i32[][])  [unwired: 2 in]
                n281 = Index Array(array=w337, index (row) #1=w341, index (col) #1=0 ("禁用的索引 (列)"), index (row) #2=w341, index (col) #2=1 ("禁用的索引 (列)")) -> (element #1=w350:i32, element #2=w351:i32)
                n282 = local read "TBD num"() -> (w333:dbl)
                n283 = local read "in TBD"() -> (w336:bool)
                n284 = local write "细胞坐标数组(X,Y)"(w337) -> ()
                n285 = call "MOV_XY_transform.vi"("error in"=w349, "芯片角点坐标"=w347, "y index"=w351, "x index"=w350) -> ("error out"=w348:errorcluster, "Y当前位置(mm)"=w343:dbl, "X当前位置(mm)"=w344:dbl, "Y实际坐标数"=w345:i32, "X实际坐标数"=w346:i32)  [unwired: 1 in]
                n286 = Increment(x=w333) -> (x+1=w334:dbl)
                n287 = local write "x pose"(w344) -> ()
                n288 = local write "y pose"(w343) -> ()
                n289 = local write "xn"(w346) -> ()
                n290 = local write "yn"(w345) -> ()
                n291 = Select(t=w333, s=w336, f=w334) -> (s? t:f=w335:dbl)
                n292 = local write "TBD num"(w335) -> ()
              }
            }
          }
          event "in TBD": Value Change {
            n293 = event-data() -> ()  [unwired: 1 in, 6 out]
            n294 = local read "in TBD"() -> (w355:bool)
            n295 = case shown="True" w355 {
              frame False {
                n296 = local write "TBD num"(0.0 ("待定数")) -> ()
              }
              frame True {
                n297 = local write "in TBD"(FALSE ("进入待定区")) -> ()
              }
            }
          }
          event "Reset": Value Change {
            n298 = event-data() -> ()  [unwired: 1 in, 6 out]
            n299 = local read "备份细胞坐标数组(X,Y)"() -> (w362:i32[][])
            n300 = local write "TBD num"(0.0 ("待定数量")) -> ()
            n301 = Array Size(array=w362) -> (size(s)=w361:i32[])
            n302 = local write "细胞坐标数组(X,Y)"(w362) -> ()
            n303 = Index Array(array=w361, index=0) -> (element=w359:i32)
            n304 = local write "Cell num"(w359) -> ()
            n305 = property on="index(1~n)" class="DigNum (strict)"("Maximum"=w359) -> ()  [unwired: 2 in, 2 out]
          }
          event "Offste/V", "Scanner", "slice par stack", "step/um": Value Change {
            w366 = T2 3 items=["no dialog", "OK message", "continue or stop message", "OK message + warnings", "continue/stop + warnings"] ("type of dialog (OK msg:1)")
            n306 = event-data() -> ()  [unwired: 1 in, 6 out]
            n307 = local read "Scanner"() -> (w390:dbl)
            n308 = local read "slice par stack"() -> (w380:dbl)
            n309 = local read "step/um"() -> (w388:dbl)
            n310 = local read "Offste/V"() -> (w383:dbl)
            n311 = call-poly <vilib>:"DAQmx Create Virtual Channel.vi"("maximum value"=10.0, "minimum value"=-10.0, "physical channels"=tag "cDAQ1Mod1/ao2") -> ("task out"=w374:refnum<k21>, "error out"=w375:errorcluster)  [unwired: 11 in]
            n312 = Divide(x=w390, y=100.0) -> (x/y=w384:dbl)
            n313 = Multiply(x=w388, y=0.024) -> (x*y=w386:dbl)
            n314 = Decrement(x=w380) -> (x-1=w379:dbl)
            n315 = local read "Offste/V"() -> (w378:dbl)
            n316 = call <vilib>:"DAQmx Start Task.vi"("task/channels in"=w374, "error in"=w375) -> ("task out"=w376:refnum<k21>, "error out"=w377:errorcluster)  [unwired: 12 in]
            n317 = Multiply(x=w386, y=w379) -> (x*y=w385:dbl)
            n318 = call-poly <vilib>:"DAQmx Write.vi"("task/channels in"=w376, "data"=w378, "error in"=w377) -> ("task out"=w370:refnum<k21>, "error out"=w369:errorcluster)  [unwired: 10 in, 1 out]
            n319 = Multiply(x=w385, y=w384) -> (x*y=w382:dbl)
            n320 = Add(x=w382, y=w383) -> (x+y=w381:dbl)
            n321 = call-poly <vilib>:"DAQmx Write.vi"("task/channels in"=w370, "data"=w381, "error in"=w369) -> ("task out"=w364:refnum<k21>, "error out"=w363:errorcluster)  [unwired: 10 in, 1 out]
            n322 = call <vilib>:"DAQmx Stop Task.vi"("task/channels in"=w364, "error in"=w363) -> ("task out"=w365:refnum<k21>, "error out"=w368:errorcluster)  [unwired: 12 in]
            n323 = call <vilib>:"DAQmx Clear Task.vi"("task in"=w365, "error in"=w368) -> ("error out"=w367:errorcluster)  [unwired: 13 in]
            n324 = call <vilib>:"Simple Error Handler.vi"("type of dialog (OK msg:1)"=w366, "error in (no error)"=w367) -> ()  [unwired: 3 in, 5 out]
          }
          event "finish": Value Change {
            n325 = event-data() -> ()  [unwired: 1 in, 6 out]
            n326 = local read "Chanber num"() -> (w393:dbl)
            n327 = local read "Cell num"() -> (w392:i32)
            n328 = local read "细胞坐标数组(X,Y)"() -> (w397:i32[][])
            n329 = Less Or Equal?(x=w393, y=w392) -> (x <= y?=w394:bool)
            n330 = Select(t=w393, s=w394, f=w392) -> (s? t:f=w391:dbl)
            n331 = local write "Chanber num"(w391) -> ()
            n332 = for {
              N: w391 -> [_]
              tunnel: w397 -> [w406] mode=indexing
              tunnel: [w401] -> w396 mode=indexing
              n333 = Index Array(array=w406, index #1=0 ("index"), index #2=1 ("index")) -> (element #1=w405:i32, element #2=w402:i32)
              n334 = Multiply(x=100, y=w405) -> (x*y=w403:i32)
              n335 = Add(x=w403, y=w402) -> (x+y=w401:i32)
            }
            n336 = local write "running"(TRUE ("running")) -> ()
            n337 = Sort 1D Array(array=w396) -> (sorted array=w395:i32[])
          }
          event "scan test": Value Change {
            (unwired) 5.0 ("荧光帧率/Hz")
            (unwired) 1.0 ("Volume number")
            n338 = event-data() -> ()  [unwired: 1 in, 6 out]
            n339 = local read "Frame rate/Hz"() -> (w410:dbl)
            n340 = local read "Volume num"() -> (w409:dbl)
            n341 = local read "slice par stack"() -> (w414:dbl)
            n342 = local read "step/um"() -> (w415:dbl)
            n343 = local read "Offste/V"() -> (w416:dbl)
            n344 = local read "Offset2/V"() -> (w412:dbl)
            n345 = call "SW-Timed_brightfield.vi"("Flip Z"=FALSE, "偏置电压"=w412, "扫描起始电压"=w416, "明场周期"=0.0, "振镜步长/um"=w415, "荧光帧率/Hz"=w410, "Image number"=w414, "Volume number"=w409) -> ()  [unwired: 4 in]
          }
        }
      }
    }
  }
  n346 = Array Size(array=w1) -> (size(s)=w40:i32[])
  n347 = Index Array(array=w40, index=0 ("索引")) -> (element=w33:i32)
  "Cell num" <- w33
  n348 = property on="index(1~n)" class="DigNum (strict)"("Maximum"=w33) -> ()  [unwired: 2 in, 2 out]
  n349 = while {
    tunnel: w30 -> [w421]
    tunnel: w29 -> [w422]
    tunnel: [w420] -> w27
    tunnel: [w419] -> w26
    tunnel: [FALSE] -> w25
    i -> [w425]
    stop <- w419 stop-if-true
    n350 = for {
      tunnel: w422 -> [w437] mode=indexing
      tunnel: w421 -> [w453]
      tunnel: [w440] -> w420
      i -> [w433]
      n351 = local read "芯片角点坐标"() -> (w452:T1)
      n352 = Quotient & Remainder(x=w437, y=100) -> (x-y*floor(x/y)=w434:i32, floor(x/y)=w435:i32)
      n353 = Increment(x=w433) -> (x+1=w432:i32)
      n354 = local write "index(1~n)"(w432) -> ()
      n355 = call "MOV_XY_transform.vi"("error in"=w453, "芯片角点坐标"=w452, "y index"=w434, "x index"=w435) -> ("error out"=w449:errorcluster, "Y当前位置(mm)"=w450:dbl, "X当前位置(mm)"=w451:dbl, "Y实际坐标数"=w438:i32, "X实际坐标数"=w439:i32)  [unwired: 1 in]
      n356 = local write "x pose"(w451) -> ()
      n357 = local write "y pose"(w450) -> ()
      n358 = local write "xn"(w439) -> ()
      n359 = local write "yn"(w438) -> ()
      n360 = flat-sequence {
        tunnel: w449 -> [w456]
        tunnel: [w455] -> w440
        frame #0 {
          w454 = T2 2 items=["no dialog", "OK message", "continue or stop message", "OK message + warnings", "continue/stop + warnings"] ("type of dialog (OK msg:1)")
          n361 = local read "Interval/ms"() -> (w457:dbl)
          n362 = Wait (ms)(milliseconds to wait=w457) -> ()  [unwired: 1 out]
          n363 = call <vilib>:"General Error Handler.vi"("type of dialog (OK msg:1)"=w454, "error in (no error)"=w456) -> ("error out"=w455:errorcluster)  [unwired: 9 in, 4 out]
        }
      }
      n364 = local read "slice par stack"() -> (w445:dbl)
      n365 = local read "Frame rate/Hz"() -> (w444:dbl)
      n366 = local read "Volume num"() -> (w446:dbl)
      n367 = local read "Offset2/V"() -> (w443:dbl)
      n368 = local read "step/um"() -> (w447:dbl)
      n369 = local read "Offste/V"() -> (w448:dbl)
      n370 = call "SW-Timed_brightfield.vi"("Flip Z"=FALSE, "偏置电压"=w443, "扫描起始电压"=w448, "明场周期"=0.0, "振镜步长/um"=w447, "error in (no error)"=w440, "荧光帧率/Hz"=w444, "Image number"=w445, "Volume number"=w446) -> ()  [unwired: 3 in]
    }
    n371 = local read "Repeat"() -> (w431:dbl)
    n372 = Decrement(x=w431) -> (x-1=w430:dbl)
    n373 = Less Or Equal?(x=w430, y=w425) -> (x <= y?=w423:bool)
    n374 = case shown="True" w423 {
      frame False {
      }
      frame True {
        n375 = local read "Period/min"() -> (w462:dbl)
        n376 = Multiply(x=w462, y=60000.0) -> (x*y=w463:dbl)
        n377 = Wait (ms)(milliseconds to wait=w463) -> ()  [unwired: 1 out]
      }
    }
    n378 = local read "Repeat 2"() -> (w429:dbl)
    n379 = local read "Repeat"() -> (w428:dbl)
    n380 = Add(x=w429, y=w428) -> (x+y=w427:dbl)
    n381 = Decrement(x=w427) -> (x-1=w426:dbl)
    n382 = Less Or Equal?(x=w426, y=w425) -> (x <= y?=w419:bool)
    n383 = Not(x=w419) -> (.not. x?=w424:bool)
    n384 = And(x=w423, y=w424) -> (x .and. y?=w417:bool)
    n385 = case shown="True" w417 {
      frame False {
      }
      frame True {
        n386 = local read "Period 2/min"() -> (w459:dbl)
        n387 = Multiply(x=w459, y=60000.0) -> (x*y=w460:dbl)
        n388 = Wait (ms)(milliseconds to wait=w460) -> ()  [unwired: 1 out]
      }
    }
  }
  n389 = local write "running"(w25) -> ()
  n390 = local write "finish"(w26) -> ()
  n391 = call "Close connection if open.vi"("System no."=1, "error in"=w27) -> ()  [unwired: 1 in, 17 out]
  "running" <- FALSE ("running")
  "finish" <- FALSE ("finish")
